vi "Has ID.vi"(8 "error in (no error)":errorcluster, 11 "Response in":refnum<class "Response.lvclass">) -> (0 "error out":errorcluster, 2 "has id?":bool, 3 "Response out":refnum<class "Response.lvclass">)   [LabVIEW 2015, in "Response.lvclass"]
uses:
  Response.lvclass
  Response.lvclass/Response.ctl
  id/id.lvclass
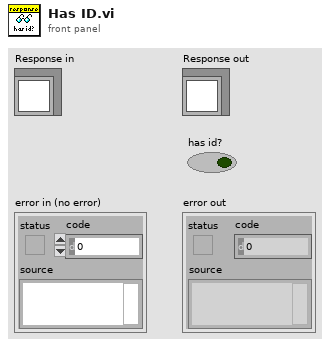
[diagram p1: front panel]
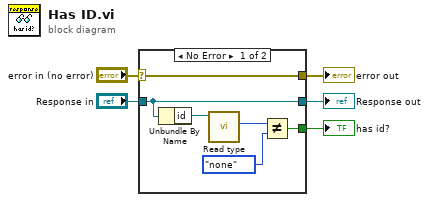
[diagram p0: block diagram]
diagram:
  n1 = case shown="No Error" "error in (no error)" {
    selector: "error in (no error)" -> [w11 w13]
    tunnel: [w11 w13] -> w4
    tunnel: [w10 w12] -> w2
    tunnel: "Response in" -> [w10 w12]
    tunnel: [w6 _] -> w1
    frame No Error {
      n2 = Unbundle By Name(w10) -> ("id"=w7:refnum<class "id.lvclass">)
      n3 = call-dynamic "Read type.vi"("id in"=w7) -> ("type"=w9:enum16{"none", "String", "Number", "NULL"})  [unwired: 8 in, 2 out]
      n4 = Not Equal?(x=w9, y=enum16{"none", "String", "Number", "NULL"}."none") -> (x != y?=w6:bool)
    }
    frame Error {
    }
  }
  "error out" <- w4
  "Response out" <- w2
  "has id?" <- w1
